vi "TP_Example.vi"() -> ()   [LabVIEW 2020]
panel:
  out "ET 4":i32
  out "Q 4":bool
  in  "Data":cluster{"Memory bit":bool, "Memory Time":i32}
  in  "Trigger":bool
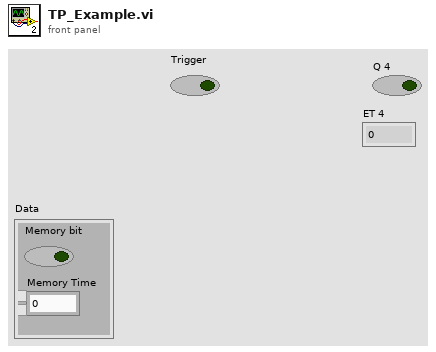
[diagram p1: front panel]
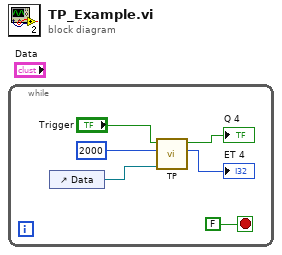
[diagram p0: block diagram]
diagram:
  n1 = while {
    stop <- FALSE stop-if-true
    n2 = control-ref of="Data"() -> (w1:refnum<vi>)
    n3 = call "TP.vi"("Cluster in"=w1, "Time"=2000, "Trigger"="Trigger") -> ("ET 4"=→"ET 4":i32, "Q 4"=→"Q 4":bool)  [unwired: 7 in]
  }
